vi "AKIP_output_on_off.vi"(8 "error in (no error)":errorcluster, 10 "Enum":enum16{"On", "Off"}(ring)=enum."Off", 11 "VISA Refnum in":refnum<visa-resource-name>="AKIP") -> (0 "error out":errorcluster, 3 "VISA Refnum out":refnum<visa-resource-name>)   [LabVIEW 2017]
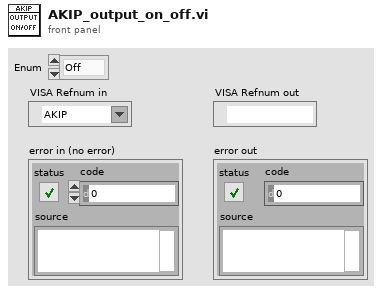
[diagram p1: front panel]
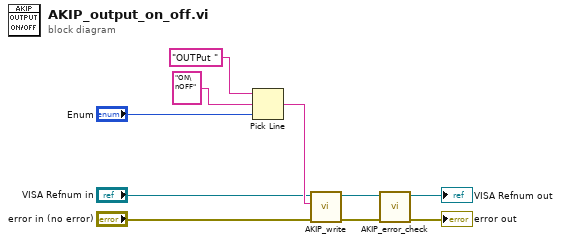
[diagram p0: block diagram]
diagram:
  n1 = Pick Line(string ("")="OUTPut " ("write buffer"), multi-line string="ON\nOFF" ("write buffer"), line index="Enum") -> (output string=w8:string)
  n2 = call "AKIP_write.vi"("error in (no error)"="error in (no error)", "write buffer"=w8, "VISA Refnum in"="VISA Refnum in") -> ("error out"=w2:errorcluster, "VISA Refnum out"=w1:refnum<visa-resource-name>)  [unwired: 7 in]
  n3 = call "AKIP_error_check.vi"("error in (no error)"=w2, "VISA Refnum in"=w1) -> ("error out"=→"error out":errorcluster, "VISA Refnum out"=→"VISA Refnum out":refnum<visa-resource-name>)  [unwired: 8 in]
